vi "Trimmed Measurement to Measurement Data.vi"(8 "Error In":errorcluster, 9 "Measurement Keys":string[](array[string]), 10 "Trimmed Worksheet Data":string[][](array[string]), 11 "NI Generic Parser in":refnum<class "NI Generic Parser.lvclass">) -> (0 "Error Out":errorcluster, 2 "Measurements From Work Sheet":T1[](array[typedef]), 3 "NI Generic Parser out":refnum<class "NI Generic Parser.lvclass">)   [LabVIEW 2016, in "NI Generic Parser.lvlib" / "NI Generic Parser.lvclass"]
uses:
  NI Generic Parser.lvclass
  Plugins/File Parsing Interface.lvlibp/Controls/Parsed Measurement.ctl
  Plugins/Measurement Data.lvlibp/Measurement Data.lvclass
  Plugins/String Database.lvlibp/String Database.lvclass
  NI Generic Parser.lvclass/NI Generic Parser.ctl
  Protected Methods/Read Measurement Description Dictionary.vi
  Support/Step Sequence Database/Multi Step Database.lvclass
  Plugins/File Parsing Interface.lvlibp/File Parsing Interface.lvclass
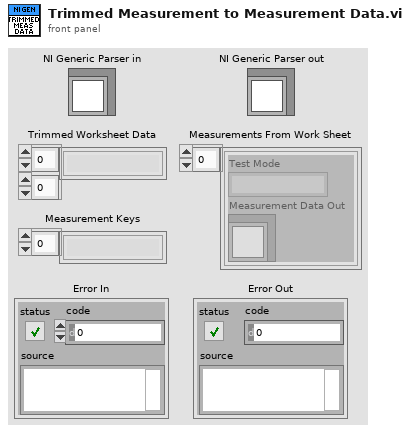
[diagram p1: front panel]
types:
  T1 = typedef "File Parsing Interface.lvlibp/File Parsing Interface.lvclass/Parsed Measurement.ctl" = cluster{"Test Mode":string, "Measurement Data Out":refnum<class "Measurement Data.lvclass">}
  T2 = typedef "Measurement Data.lvlibp/Measurement Data.lvclass/Measurement Description.ctl" = cluster{"Measurement Sequence Position":T3, "Measurement Data":refnum<class "String Database.lvclass">, "Measurement Definition Entry":string}
  T3 = typedef "Measurement Data.lvlibp/Measurement Data.lvclass/Measurement Position.ctl" = enum16{"PreMeasurement", "MainMeasurement", "PostMeasurement"}
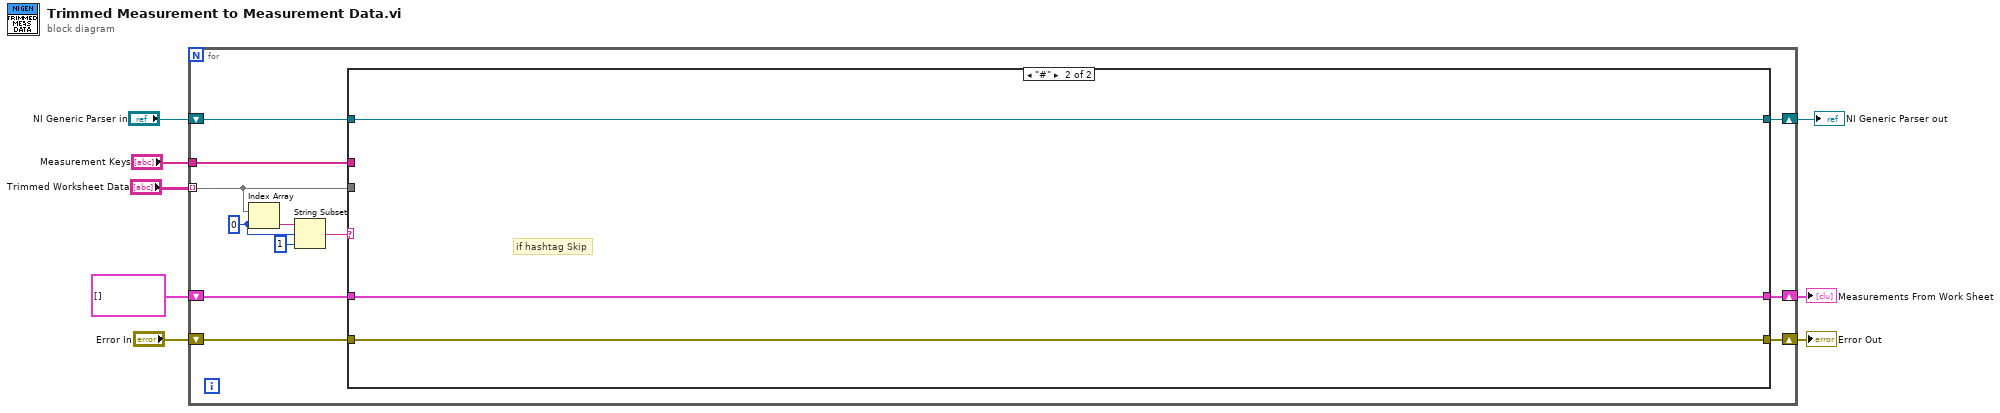
[diagram p0: block diagram]
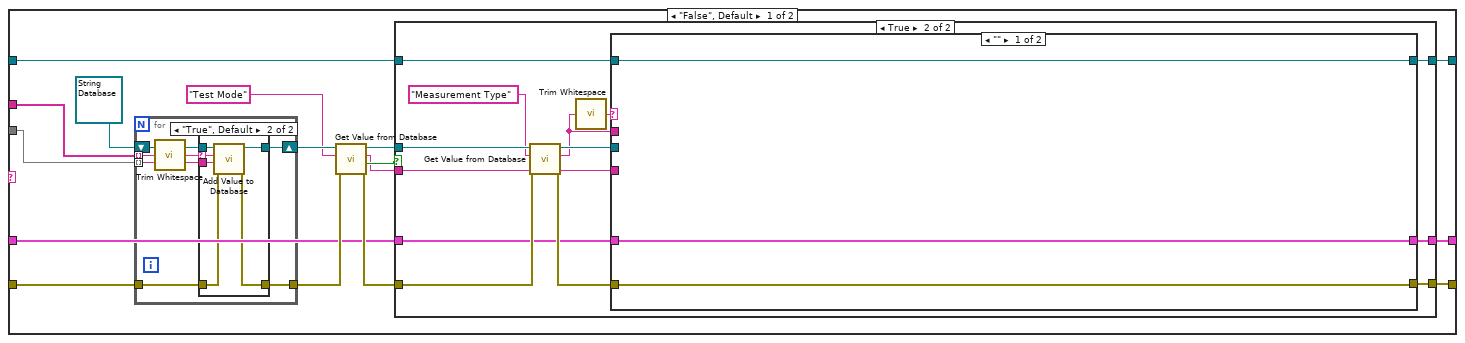
[diagram p2: hidden frame]
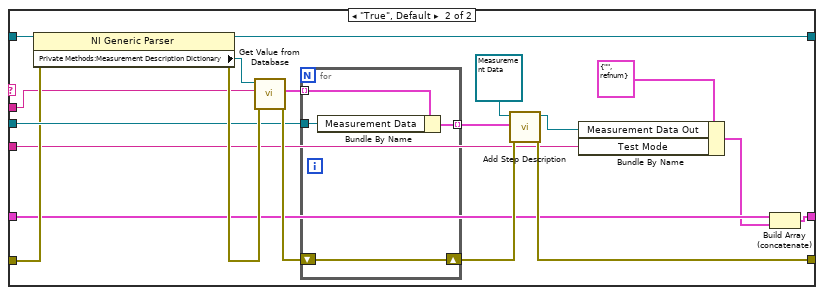
[diagram p4: hidden frame]
diagram:
  n1 = for {
    tunnel: "Trimmed Worksheet Data" -> [w14] mode=indexing
    tunnel: "Measurement Keys" -> [w13]
    shift-right: [w15] -> w8
    shift-left: "NI Generic Parser in" -> [w16]
    shift-right: [w20] -> w3
    shift-left: "Error In" -> [w19]
    shift-right: [w11] -> w1
    shift-left: T1[] [] -> [w10]
    w12 = 0 ("index")
    n2 = Index Array(array=w14, index=w12) -> (element=w18:string)
    n3 = String Subset(string=w18, offset (0)=w12, length (rest)=1 ("length (rest)")) -> (substring=w17:string)
    n4 = case shown="\"#\"" w17 {
      tunnel: [w27 w96] -> w20
      tunnel: w19 -> [w35 w96]
      tunnel: w16 -> [w29 w95]
      tunnel: [w28 w95] -> w15
      tunnel: w14 -> [w33 _]
      tunnel: w13 -> [w34 _]
      tunnel: [w23 w94] -> w11
      tunnel: w10 -> [w24 w94]
      frame "False", Default {
        n5 = for {
          tunnel: [w84] -> w31
          tunnel: w35 -> [w83]
          tunnel: w34 -> [w82] mode=indexing
          shift-right: [w80] -> w32
          shift-left: refnum<class "String Database.lvclass"> refnum ("String Database.lvlibp:String Dictionary") -> [w85]
          tunnel: w33 -> [w81] mode=indexing
          n6 = call <vilib>:"Trim Whitespace.vi"("string"=w82) -> ("trimmed string"=w79:string)  [unwired: 1 in]
          n7 = case shown="\"True\", Default" w79 {
            selector: w79 -> [_ w90]
            tunnel: w85 -> [w87 w93]
            tunnel: [w86 w92] -> w84
            tunnel: w83 -> [w86 w91]
            tunnel: w81 -> [_ w89]
            tunnel: [w87 w88] -> w80
            frame "" {
            }
            frame "True", Default {
              n8 = call "Add Value to Database.vi"("error in (no error)"=w91, "Entry Value"=w89, "Entry Name"=w90, "Dictionary In"=w93) -> ("error out"=w92:errorcluster, "Dictionary Out"=w88:refnum<class "String Database.lvclass">)  [unwired: 5 in, 1 out]
            }
          }
        }
        n9 = call "Get Value from Database.vi"("error in (no error)"=w31, "Entry Name"="Test Mode", "Message in"=w32) -> ("error out"=w25:errorcluster, "Entry Found"=w22:bool, "Entry Value"=w21:string, "Message out"=w26:refnum<class "String Database.lvclass">)  [unwired: 5 in]
        n10 = case shown="True" w22 {
          tunnel: w29 -> [w37 w52]
          tunnel: [w37 w51] -> w28
          tunnel: [w38 w50] -> w27
          tunnel: w26 -> [_ w49]
          tunnel: w25 -> [w38 w47]
          tunnel: w24 -> [w39 w44]
          tunnel: [w39 w43] -> w23
          tunnel: w21 -> [_ w42]
          frame False {
          }
          frame True {
            n11 = call "Get Value from Database.vi"("error in (no error)"=w47, "Entry Name"="Measurement Type", "Message in"=w49) -> ("error out"=w46:errorcluster, "Entry Value"=w41:string, "Message out"=w48:refnum<class "String Database.lvclass">)  [unwired: 5 in, 1 out]
            n12 = call <vilib>:"Trim Whitespace.vi"("string"=w41) -> ("trimmed string"=w40:string)  [unwired: 1 in]
            n13 = case shown="\"\"" w40 {
              tunnel: w52 -> [w53 w74]
              tunnel: [w53 w73] -> w51
              tunnel: [w55 w65] -> w50
              tunnel: w48 -> [_ w64]
              tunnel: w46 -> [w55 w63]
              tunnel: w44 -> [w54 w61]
              tunnel: [w54 w60] -> w43
              tunnel: w42 -> [_ w58]
              tunnel: w41 -> [_ w56]
              frame "" {
              }
              frame "True", Default {
                n14 = property class="NI Generic Parser"(reference=w74, error in=w63) -> (reference out=w73:refnum<class "NI Generic Parser.lvclass">, error out=w71:errorcluster, "Private Methods:Measurement Description Dictionary"=w72:refnum<class "Multi Step Database.lvclass">)
                n15 = call "Get Value from Database.vi"("error in (no error)"=w71, "Measurement Name"=w56, "Multi Step Database in"=w72) -> ("error out"=w70:errorcluster, "Measurement Definition"=w69:T2[])  [unwired: 6 in, 1 out]
                n16 = for {
                  tunnel: w64 -> [w76]
                  shift-right: [w78] -> w66
                  shift-left: w70 -> [w78]
                  tunnel: w69 -> [w77] mode=indexing
                  tunnel: [w75] -> w67 mode=indexing
                  n17 = Bundle By Name(cluster=w77, "Measurement Data"=w76) -> (w75:T2)
                }
                n18 = call "Add Step Description.vi"("error in (no error)"=w66, "New Step Description"=w67, "Measurement Data in"=refnum<class "Measurement Data.lvclass"> refnum ("Measurement Data.lvlibp:Measurement Data")) -> ("error out"=w65:errorcluster, "Measurement Data out"=w62:refnum<class "Measurement Data.lvclass">)  [unwired: 7 in]
                n19 = Bundle By Name(cluster=T1 {"Test Mode"="", "Measurement Data Out"=refnum} ("Cluster"), "Measurement Data Out"=w62, "Test Mode"=w58) -> (w59:T1)
                n20 = Build Array (concatenate)(w61, w59) -> (w60:T1[])
              }
            }
          }
        }
      }
      frame "#" {
        # "if hashtag Skip"
      }
    }
  }
  "NI Generic Parser out" <- w8
  "Error Out" <- w3
  "Measurements From Work Sheet" <- w1
